vi "GlobalControlVariables.vi"() -> ()   [LabVIEW 2016]
panel:
  out "Data Read Timeout (ms)":u32=25
  out "Analog Format":string="%5.3f"
  out "Ready Read End (ms)":u32
  out "Ready Read Wait (ms)":u32=500
  out "TCP Digital Array":u32[](array[numeric])
  out "CloseSubVIs":bool
  out "TCP Analog Array":dbl[](array[numeric])
  out "Data Update Wait (ms)":u32=100
  out "GUI Update Wait (ms)":u32=250
  out "Date Write Wait (ms)":u32=25
  out "Data Read Wait (ms)":u32=25
  out "TCP Write Sema":T1
  out "TCP Read Data":string
  out "TCP Ready Read":bool
  out "Global Error Message":string
  out "TPC Write Sema Name":string="TCP Sema"
  out "TCP Write Data":string
  out "Quit":bool
  in  "TCP error":errorcluster
  out "Default Port":u16=3306
  in  "TCP Refnum":refnum<k5>
  out "Connected?":bool
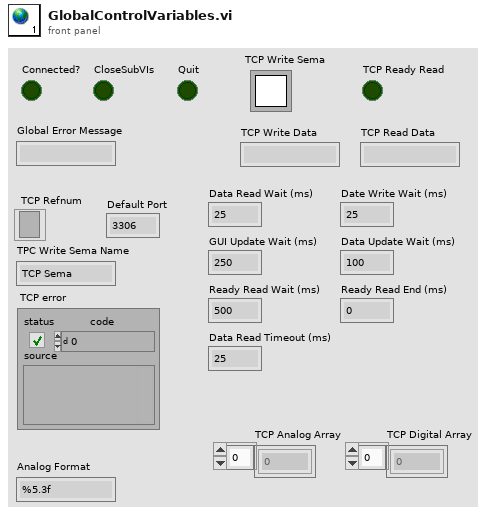
[diagram p1: front panel]
types:
  T1 = typedef "Semaphore RefNum" = refnum<k1>
diagram:
